vi "Conversor Celcius Fahrenheit.vi"() -> ()   [LabVIEW 2022 SP3]
panel:
  in  "Tf":dbl
  in  "Tc":dbl
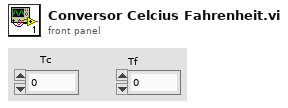
[diagram p1: front panel]
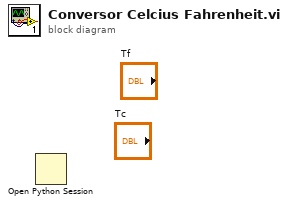
[diagram p0: block diagram]
diagram:
  n1 = Open Python Session() -> ()  [unwired: 3 in, 2 out]
